vi "GFV project info.vi"(1 "Action(GET)":enum16{"GET", "SET"}(ring), 7 "Project info in":T1, 11 "error in (no error)":errorcluster) -> (8 "Project info out":T1, 15 "error out":errorcluster)   [LabVIEW 2011]
uses:
  Project infor with project path.ctl
  Project in icluster.ctl
  GUI/Job setup/Job and site cluster.ctl
  emi cndiates/List of all contrys(combo box).ctl
  GUI/Job setup/Tool registration ID.ctl
  Run Information.ctl
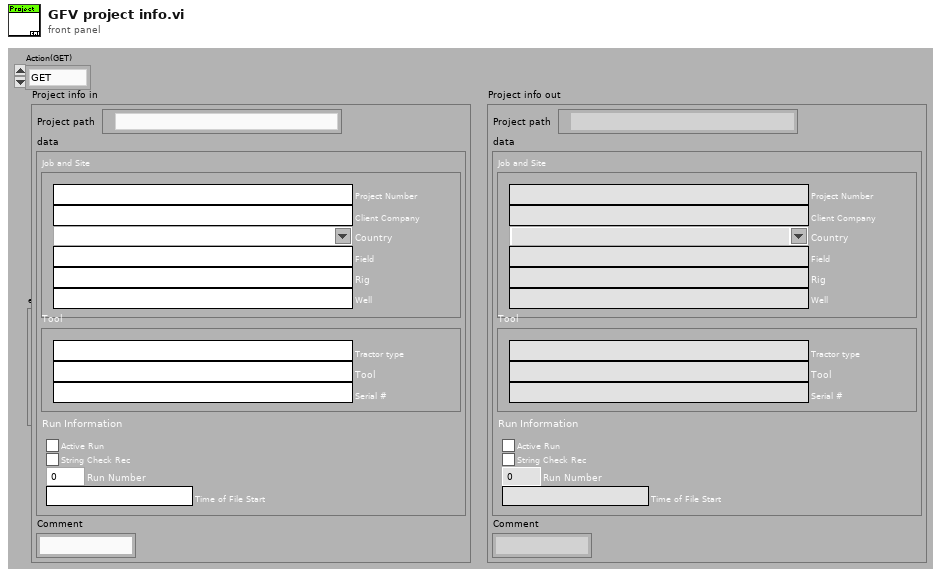
[diagram p1: front panel]
types:
  T1 = typedef "Project infor with project path.ctl" = cluster{"Project path":path, "data":T2, "Comment":string}
  T2 = typedef "Project in icluster.ctl" = cluster{"Job and Site":T3, "Tool":T5, "Run Information":T6}
  T3 = typedef "Job and site cluster.ctl" = cluster{"Project Number":string, "Client Company":string, "Country":T4, "Field":string, "Rig":string, "Well":string}
  T4 = typedef "List of all contrys(combo box).ctl" = string
  T5 = typedef "Tool registration ID.ctl" = cluster{"Tractor type":string, "Tool":string, "Serial #":string}
  T6 = typedef "Run Information.ctl" = cluster{"Active Run":bool, "String Check Rec":bool, "Run Number":i32, "Time of File Start":string}
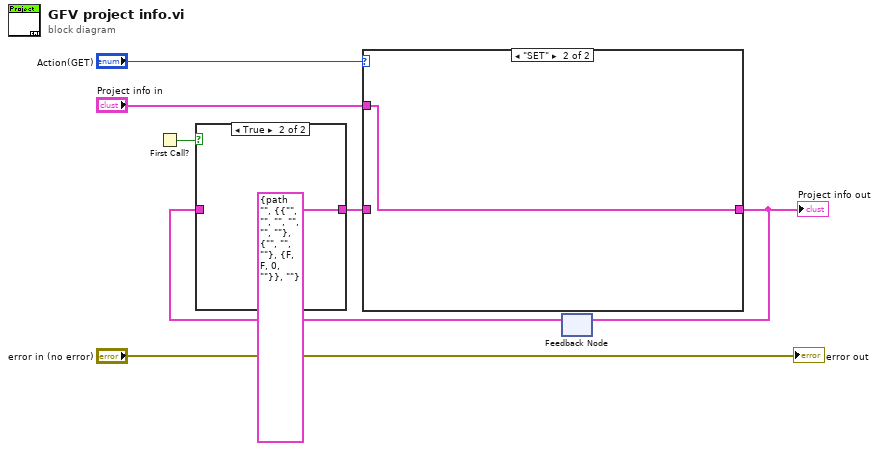
[diagram p0: block diagram]
diagram:
  n1 = First Call?() -> (First Call?: T/F=w4:bool)
  n2 = feedback #1() -> (w5:T1)  [unwired: 1 in]
  n3 = case shown="True" w4 {
    tunnel: w5 -> [w8 _]
    tunnel: [w8 T1 {"Project path"=path "", "data"={"Job and Site"={"Project Number"="", "Client Company"="", "Country"="", "Field"="", "Rig"="", "Well"=""}, "Tool"={"Tractor type"="", "Tool"="", "Serial #"=""}, "Run Information"={"Active Run"=FALSE, "String Check Rec"=FALSE, "Run Number"=0, "Time of File Start"=""}}, "Comment"=""} ("Project info")] -> w2
    frame False {
    }
    frame True {
    }
  }
  n4 = case shown="\"SET\"" "Action(GET)" {
    tunnel: [w10 w11] -> w3
    tunnel: w2 -> [w10 _]
    tunnel: "Project info in" -> [_ w11]
    frame "GET", Default {
    }
    frame "SET" {
    }
  }
  "Project info out" <- w3
  n5 = feedback-in #1(w3) -> ()
  "error out" <- "error in (no error)"
